vi "MIC_OUT.vi"() -> ()   [LabVIEW 2018]
uses:
  <vilib>/DAQmx/write.llb/DAQmx Write (Analog Wfm 1Chan NSamp).vi
  <vilib>/DAQmx/create/channels.llb/DAQmx Create Channel (AO-Voltage-Basic).vi
  <vilib>/DAQmx/configure/timing.llb/DAQmx Timing (Use Waveform).vi
  <vilib>/DAQmx/miscellaneous.llb/DAQmx Fill In Error Info.vi
panel:
  in  "y":bool
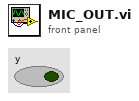
[diagram p1: front panel]
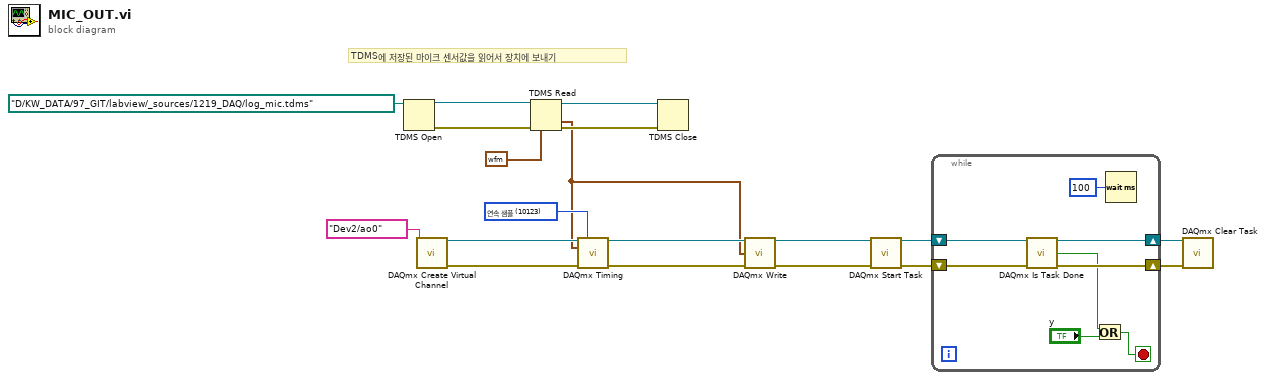
[diagram p0: block diagram]
diagram:
  w8 = 10123 items=["유한 샘플"=10178, "연속 샘플"=10123, "하드웨어 타이밍에 의한 단일 포인트"=12522] ("sample mode")
  # "TDMS에 저장된 마이크 센서값을 읽어서 장치에 보내기"
  n1 = TDMS Open(11:path "D:/KW_DATA/97_GIT/labview/_sources/1219_DAQ/log_mic.tdms" ("파일 경로")) -> (0:w6:errorcluster, 3:w7:refnum<k34>)  [unwired: 6 in]
  n2 = call-poly <vilib>:"DAQmx Create Virtual Channel.vi"("physical channels"=tag "Dev2/ao0") -> ("task out"=w19:refnum<k21>, "error out"=w18:errorcluster)  [unwired: 13 in]
  n3 = TDMS Read(0:w7, 11:w6, 12:waveform(dbl) {"t0"=timestamp(0 s since 1904-01-01), "dt"=0.0, "Y"=[]} ("waveform")) -> (4:w5:refnum<k34>, 10:w1:waveform(dbl), 15:w4:errorcluster)  [unwired: 5 in, 3 out]
  n4 = call-poly <vilib>:"DAQmx Timing.vi"("task/channels in"=w19, "sample mode"=w8, "waveform"=w1, "error in"=w18) -> ("task out"=w17:refnum<k21>, "error out"=w16:errorcluster)  [unwired: 10 in]
  n5 = TDMS Close(8:w4, 11:w5) -> ()  [unwired: 2 out]
  n6 = call-poly <vilib>:"DAQmx Write.vi"("task/channels in"=w17, "data"=w1, "error in"=w16) -> ("task out"=w15:refnum<k21>, "error out"=w14:errorcluster)  [unwired: 10 in, 1 out]
  n7 = call <vilib>:"DAQmx Start Task.vi"("task/channels in"=w15, "error in"=w14) -> ("task out"=w13:refnum<k21>, "error out"=w12:errorcluster)  [unwired: 12 in]
  n8 = while {
    shift-right: [w25] -> w11
    shift-left: w13 -> [w27]
    shift-right: [w24] -> w10
    shift-left: w12 -> [w26]
    stop <- w23 stop-if-true
    n9 = call <vilib>:"DAQmx Is Task Done.vi"("task/channels in"=w27, "error in"=w26) -> ("task out"=w25:refnum<k21>, "task done?"=w21:bool, "error out"=w24:errorcluster)  [unwired: 11 in]
    n10 = Or(x=w21, y="y") -> (x .or. y?=w23:bool)
    n11 = Wait (ms)(milliseconds to wait=u32 100 ("대기 시간 (ms)")) -> ()  [unwired: 1 out]
  }
  n12 = call <vilib>:"DAQmx Clear Task.vi"("task in"=w11, "error in"=w10) -> ()  [unwired: 13 in, 1 out]
